vi "Thorlabs-Update Pinhole.vi"(8 "error in (no error)":errorcluster, 11 "params":variant) -> (0 "error out":errorcluster)   [LabVIEW 2020]
uses:
  MPH_SDK/MPH16.lvlib
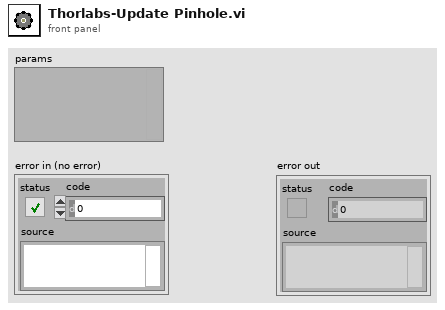
[diagram p1: front panel]
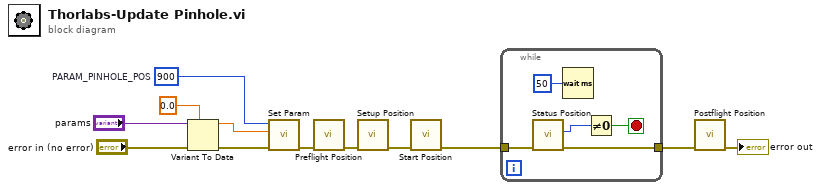
[diagram p0: block diagram]
diagram:
  w3 = 900  # PARAM_PINHOLE_POS
  n1 = Variant To Data(error in="error in (no error)", type=0.0, Variant="params") -> (data=w10:dbl, error out=w12:errorcluster)
  n2 = call "Set Param.vi"("error in (no error)"=w12, "param"=w10, "paramID"=w3) -> ("error out"=w6:errorcluster)  [unwired: 3 in, 1 out]
  n3 = call "Preflight Position.vi"("error in (no error)"=w6) -> ("error out"=w2:errorcluster)  [unwired: 5 in, 1 out]
  n4 = call "Setup Position.vi"("error in (no error)"=w2) -> ("error out"=w7:errorcluster)  [unwired: 5 in, 1 out]
  n5 = call "Start Position.vi"("error in (no error)"=w7) -> ("error out"=w5:errorcluster)  [unwired: 5 in, 1 out]
  n6 = while {
    tunnel: w5 -> [w17]
    tunnel: [w16] -> w4
    stop <- w13 stop-if-true
    n7 = call "Status Position.vi"("error in (no error)"=w17) -> ("error out"=w16:errorcluster, "function return"=w14:i32)  [unwired: 4 in, 1 out]
    n8 = Wait (ms)(milliseconds to wait=u32 50) -> ()  [unwired: 1 out]
    n9 = Not Equal To 0?(x=w14) -> (x != 0?=w13:bool)
  }
  n10 = call "Postflight Position.vi"("error in (no error)"=w4) -> ("error out"=→"error out":errorcluster)  [unwired: 5 in, 1 out]
